vi "Window Frequency Response (double Array).vi"(8 "N (window length)":i32=512, 10 "window":T1(ring), 11 "f(normalized)":dbl[](array[numeric]) format="%.5f") -> (3 "H(f)":cdb[](array[numeric]) format="%.2f")   [LabVIEW 2021]
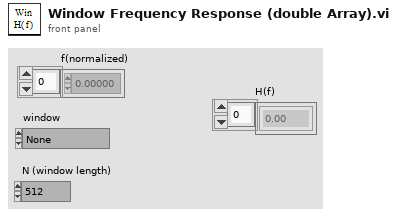
[diagram p1: front panel]
types:
  T1 = enum16{"None ", "Hanning", "Hamming", "Blackman-Harris", "Exact Blackman", "Blackman", "Flat Top", "4 Term B-Harris ", "7 Term B-Harris", "Low Sidelobe"}
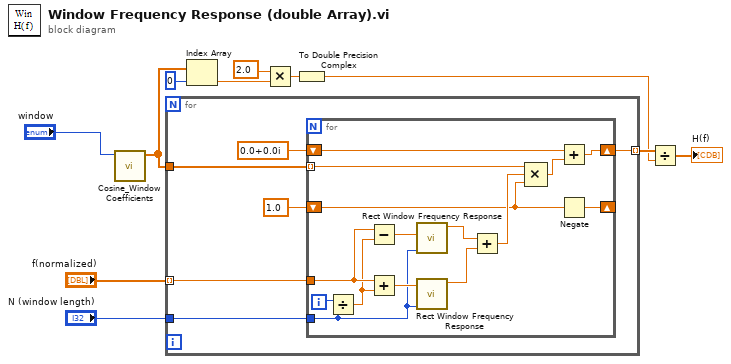
[diagram p0: block diagram]
diagram:
  n1 = call "Cosine_Window Coefficients.vi"("window"="window") -> ("WinCoefficients"=w4:dbl[])  [unwired: 10 in]
  n2 = for {
    tunnel: "f(normalized)" -> [w15] mode=indexing
    tunnel: "N (window length)" -> [w14]
    tunnel: [w13] -> w5 mode=indexing
    tunnel: w4 -> [w12]
    n3 = for {
      tunnel: w12 -> [w29] mode=indexing
      tunnel: w15 -> [w26]
      tunnel: w14 -> [w22]
      shift-right: [w30] -> w13
      shift-left: cdb 0.0+0.0i -> [w31]
      shift-right: [w19] -> _
      shift-left: 1.0 ("y") -> [w18]
      i -> [w32]
      n4 = Divide(x=w32, y=w22) -> (x/y=w25:dbl)
      n5 = Subtract(x=w26, y=w25) -> (x-y=w23:dbl)
      n6 = Add(x=w26, y=w25) -> (x+y=w24:dbl)
      n7 = call "Rect Window Frequency Response.vi"("N"=w22, "f"=w23) -> ("H(f)"=w21:cdb)  [unwired: 9 in]
      n8 = call "Rect Window Frequency Response.vi"("N"=w22, "f"=w24) -> ("H(f)"=w20:cdb)  [unwired: 9 in]
      n9 = Add(x=w21, y=w20) -> (x+y=w28:cdb)
      n10 = Compound Arithmetic op=MULTIPLY(w29, w28, w18) -> (w27:cdb)
      n11 = Add(x=w31, y=w27) -> (x+y=w30:cdb)
      n12 = Negate(x=w18) -> (-x=w19:dbl)
    }
  }
  n13 = Index Array(array=w4, index=0 ("Index")) -> (element=w7:dbl)
  n14 = Multiply(x=2.0 ("y"), y=w7) -> (x*y=w3:dbl)
  n15 = To Double Precision Complex(1:w3) -> (0:w1:cdb)
  n16 = Divide(x=w5, y=w1) -> (x/y=→"H(f)":cdb[])
